vi "LVUSBRH2_VISA_CMD_echo_onoff.vi"(8 "error in (no error)":errorcluster caption="error in(no errro)", 9 "echo on/off)(F)":bool, 11 "VISA rssc":refnum<visa-resource-name>) -> (0 "error out":errorcluster, 3 "VISA rssc out":refnum<visa-resource-name>)   [LabVIEW 2020]
uses:
  <vilib>/Instr/_visa.llb/VISA Flush IO Buffer Mask.ctl
panel:
  out "cmd string":string
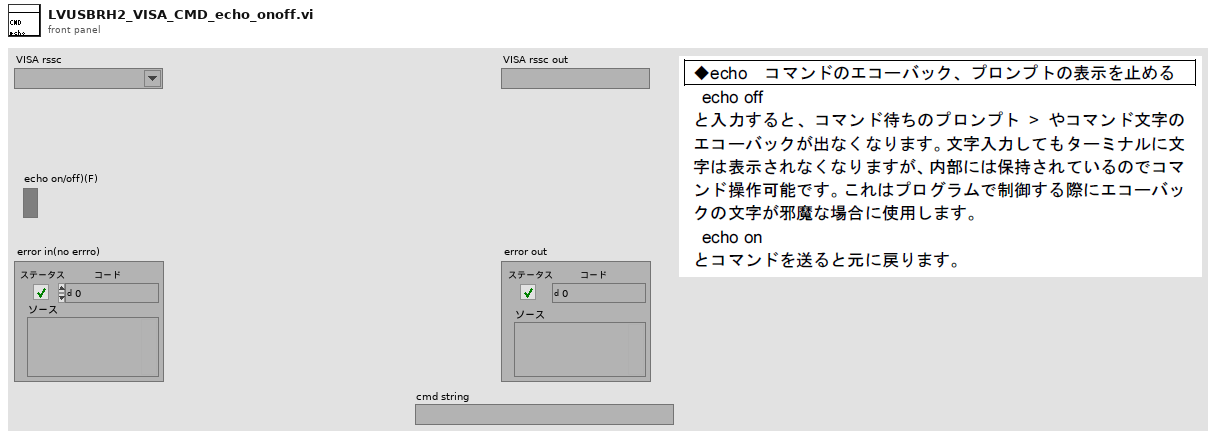
[diagram p1: front panel]
types:
  T1 = typedef "VISA Flush IO Buffer Mask.ctl" = u16
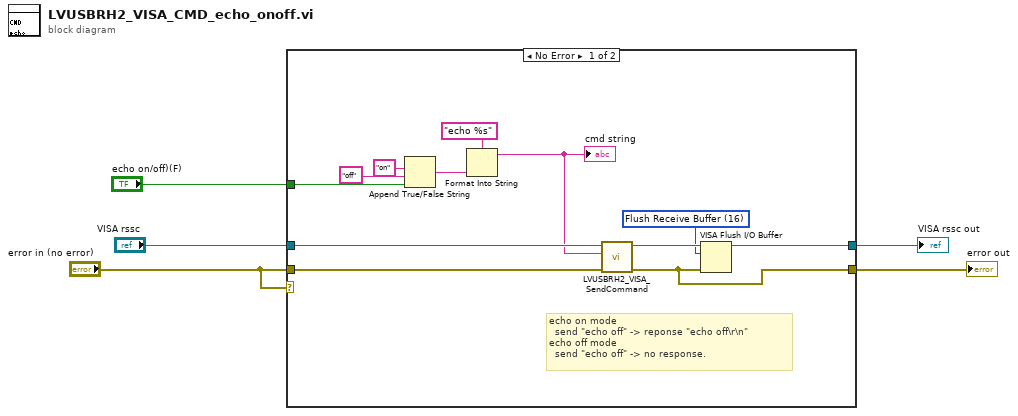
[diagram p0: block diagram]
diagram:
  n1 = case shown="No Error" "error in (no error)" {
    tunnel: "VISA rssc" -> [w17 w19]
    tunnel: [w8 w19] -> w4
    tunnel: "error in (no error)" -> [w16 w18]
    tunnel: [w7 w18] -> w3
    tunnel: "echo on/off)(F)" -> [w13 _]
    frame No Error {
      w6 = T1 16 items=["Flush Receive Buffer"=16, "Write Transmit Buffer to Device"=32, "Flush Receive Buffer (No I/O)"=64, "Flush Transmit Buffer"=128] ("Mask")
      # "echo on mode\n  send \"echo off\" -> reponse \"echo off\\r\\n\"\necho off mode\n  send \"echo off\" -> no response."
      n2 = Append True/False String(1:w13, 2:"off" ("TRUE文字列"), 3:"on" ("TRUE文字列")) -> (0:w10:string)  [unwired: 1 in]
      n3 = Format Into String(format string="echo %s" ("形式文字列"), w10) -> (resulting string=w14:string)  [unwired: 2 in, 1 out]
      "cmd string" <- w14
      n4 = call "LVUSBRH2_VISA_SendCommand.vi"("error in (no error)"=w16, "cmd string"=w14, "VISA rssc"=w17) -> ("error out"=w7:errorcluster, "VISA rssc out"=w9:refnum<visa-resource-name>)  [unwired: 7 in]
      n5 = VISA Flush I/O Buffer(VISA resource name=w9, mask (16)=w6, error in (no error)=w7) -> (VISA resource name out=w8:refnum<visa-resource-name>)  [unwired: 1 out]
    }
    frame Error {
    }
  }
  "VISA rssc out" <- w4
  "error out" <- w3
